vi "fpga_sine_KA.vi"() -> ()   [LabVIEW 2018]
uses:
  <vilib>/rvi/FXPMathLib/FxpSinAndCos/subVIs/nifxpmath_SinAndCos_SimConfig.ctl
  <vilib>/rvi/Emulation/niFpgaGetClockAttributes.vi
  <vilib>/rvi/Emulation/niFpgaSctlEmulationGetInTimedLoop.vi
  <vilib>/rvi/Emulation/niFpgaEmulationReportErrorSimple.vi
  <vilib>/rvi/FXPMathLib/FxpSinAndCos/simVIs/DllFxpSinAndCosTemp_sub.vi
  <vilib>/rvi/eio/common/nirviEmuTemplateMethod_errors.vi
  <vilib>/rvi/Emulation/niFpgaCriticalErrorInLSC.vi
  <vilib>/rvi/FXPMathLib/FxpSinAndCos/XNode/nifxpmath_SinAndCos.xnode
  <vilib>/eio/EIONode/EIONode.xnode
panel:
  out "0":i32=696
  in  "mult":fxp<+,16,-8>=0.0009999871253967285
  in  "y":i32=2000
  in  "Count(uSec)":u32=10
  out "sine out":i16=1648
  in  "offset":i16
  in  "amplitude":i16=2018
  in  "Stop Button":bool
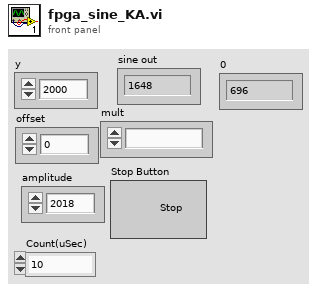
[diagram p1: front panel]
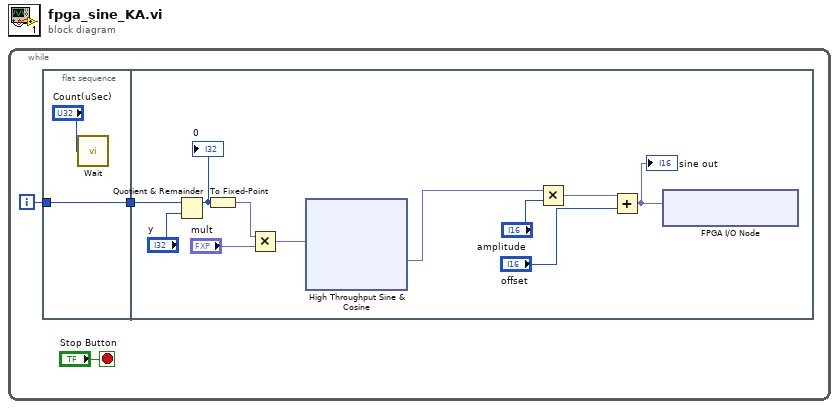
[diagram p0: block diagram]
diagram:
  n1 = while {
    i -> [w2]
    stop <- "Stop Button" stop-if-true
    n2 = flat-sequence {
      tunnel: w2 -> [w5]
      tunnel: [w5] -> w1
      tunnel: w1 -> [w11]
      frame #0 {
        n3 = call "Wait"("Count(uSec)"="Count(uSec)") -> ()  [unwired: 1 out]
      }
      frame #1 {
        n4 = Quotient & Remainder(x=w11, y="y") -> (x-y*floor(x/y)=w8:i32)  [unwired: 1 out]
        "0" <- w8
        n5 = To Fixed-Point(number=w8) -> (fixed-point=w7:fxp<+/-,16,12>)  [unwired: 1 in]
        n6 = Multiply(x=w7, y="mult") -> (x*y=w6:fxp<+/-,32,4>)
        n7 = xnode "High Throughput Sine & Cosine"("x (pi)"=w6) -> ("sin(x)"=w12:fxp<+/-,16,2>)  [unwired: 1 out]
        n8 = Multiply(x=w12, y="amplitude") -> (x*y=w15:fxp<+/-,32,18>)
        n9 = Add(x=w15, y="offset") -> (x+y=w13:fxp<+/-,32,18>)
        "sine out" <- w13
        n10 = xnode "FPGA I/O Node"("ConnectorC/AO0"=w13) -> ()  [unwired: 1 in, 1 out]
      }
    }
  }
